vi "GetPositionDegreeInc.vi"(8 "error in (no error)":errorcluster, 10 "IncImpulsIn":dbl caption="Инкремент импульсов", 11 "StepMotor in":refnum<class "StepMotor.lvclass">) -> (0 "error out":errorcluster, 2 "IncImpulsOut":dbl caption="Инкремент импульсов", 3 "StepMotor out":refnum<class "StepMotor.lvclass">)   [LabVIEW 2010, in "StepMotor.lvclass"]
uses:
  StepMotor.lvclass
panel:
  out "RawValue":dbl
  out "Текущая позиция":dbl
  out "Предыдущая позиция":dbl
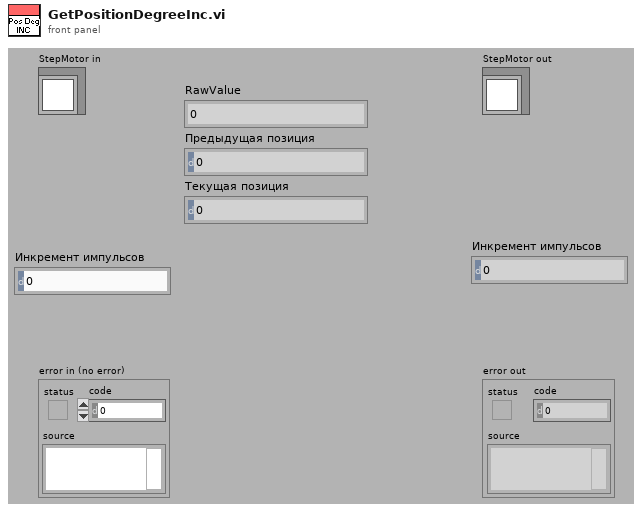
[diagram p1: front panel]
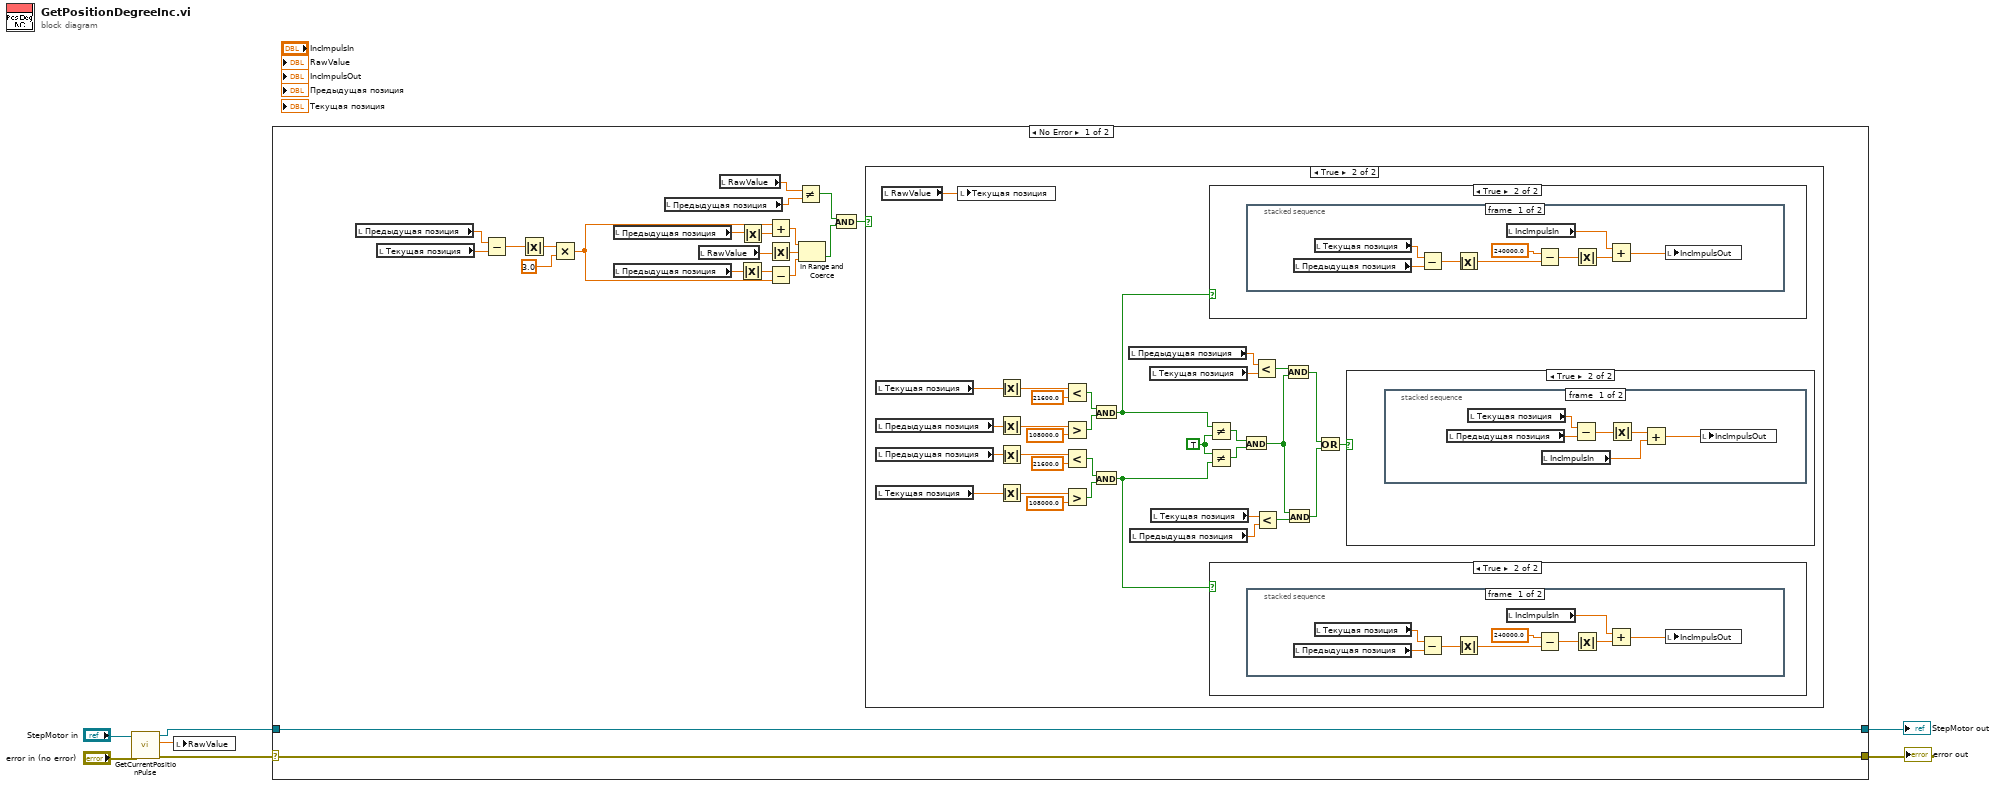
[diagram p0: block diagram]
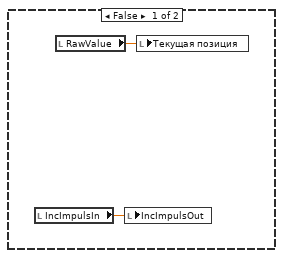
[diagram p2: hidden frame]
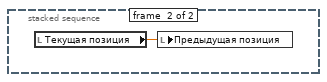
[diagram p4: hidden frame]
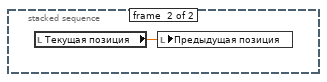
[diagram p6: hidden frame]
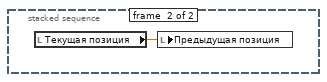
[diagram p8: hidden frame]
diagram:
  n1 = call-dynamic "GetCurrentPositionPulse.vi"("error in (no error)"="error in (no error)", "StepMotor in"="StepMotor in") -> ("error out"=w2:errorcluster, "Текущая позиция"=w5:dbl, "StepMotor out"=w1:refnum<class "StepMotor.lvclass">)  [unwired: 7 in]
  n2 = local write "RawValue"(w5) -> ()
  n3 = case shown="No Error" w2 {
    selector: w2 -> [w10 w91]
    tunnel: [w10 w91] -> w7
    tunnel: [w11 w90] -> w6
    tunnel: w1 -> [w11 w90]
    frame No Error {
      n4 = local read "Предыдущая позиция"() -> (w27:dbl)
      n5 = local read "Текущая позиция"() -> (w25:dbl)
      n6 = Subtract(x=w27, y=w25) -> (x-y=w24:dbl)
      n7 = Absolute Value(x=w24) -> (abs(x)=w22:dbl)
      n8 = Multiply(x=w22, y=3.0) -> (x*y=w28:dbl)
      n9 = local read "Предыдущая позиция"() -> (w18:dbl)
      n10 = local read "Предыдущая позиция"() -> (w17:dbl)
      n11 = local read "Предыдущая позиция"() -> (w26:dbl)
      n12 = local read "RawValue"() -> (w8:dbl)
      n13 = local read "RawValue"() -> (w9:dbl)
      n14 = Absolute Value(x=w17) -> (abs(x)=w16:dbl)
      n15 = Absolute Value(x=w18) -> (abs(x)=w19:dbl)
      n16 = Add(x=w28, y=w19) -> (x+y=w15:dbl)
      n17 = Absolute Value(x=w8) -> (abs(x)=w20:dbl)
      n18 = Subtract(x=w16, y=w28) -> (x-y=w14:dbl)
      n19 = Not Equal?(x=w9, y=w26) -> (x != y?=w13:bool)
      n20 = In Range and Coerce(upper limit=w15, x=w20, lower limit=w14) -> (In Range?=w12:bool)  [unwired: 1 out]
      n21 = Compound Arithmetic op=AND(w13, w12) -> (w23:bool)
      n22 = case shown="True" w23 {
        frame False {
          n23 = local read "IncImpulsIn"() -> (w29:dbl)
          n24 = local read "RawValue"() -> (w30:dbl)
          n25 = local write "IncImpulsOut"(w29) -> ()
          n26 = local write "Текущая позиция"(w30) -> ()
        }
        frame True {
          w54 = TRUE ("x")
          n27 = local read "Текущая позиция"() -> (w31:dbl)
          n28 = local read "Предыдущая позиция"() -> (w33:dbl)
          n29 = local read "Предыдущая позиция"() -> (w35:dbl)
          n30 = local read "Текущая позиция"() -> (w37:dbl)
          n31 = local read "RawValue"() -> (w39:dbl)
          n32 = local write "Текущая позиция"(w39) -> ()
          n33 = Absolute Value(x=w31) -> (abs(x)=w32:dbl)
          n34 = Absolute Value(x=w33) -> (abs(x)=w34:dbl)
          n35 = Absolute Value(x=w35) -> (abs(x)=w36:dbl)
          n36 = Absolute Value(x=w37) -> (abs(x)=w38:dbl)
          n37 = Less?(x=w32, y=21600.0) -> (x < y?=w57:bool)
          n38 = Greater?(x=w34, y=108000.0) -> (0:w58:bool)
          n39 = Less?(x=w36, y=21600.0) -> (x < y?=w56:bool)
          n40 = Greater?(x=w38, y=108000.0) -> (0:w55:bool)
          n41 = And(x=w57, y=w58) -> (x .and. y?=w43:bool)
          n42 = And(x=w56, y=w55) -> (x .and. y?=w42:bool)
          n43 = local read "Предыдущая позиция"() -> (w50:dbl)
          n44 = local read "Предыдущая позиция"() -> (w49:dbl)
          n45 = local read "Текущая позиция"() -> (w41:dbl)
          n46 = local read "Текущая позиция"() -> (w40:dbl)
          n47 = Not Equal?(x=w43, y=w54) -> (x != y?=w52:bool)
          n48 = Not Equal?(x=w54, y=w42) -> (x != y?=w53:bool)
          n49 = case shown="True" w43 {
            frame False {
            }
            frame True {
              n50 = stacked-sequence {
                frame #0 {
                  n51 = local read "Предыдущая позиция"() -> (w88:dbl)
                  n52 = local read "Текущая позиция"() -> (w80:dbl)
                  n53 = Subtract(x=w80, y=w88) -> (x-y=w87:dbl)
                  n54 = Absolute Value(x=w87) -> (abs(x)=w86:dbl)
                  n55 = local read "IncImpulsIn"() -> (w83:dbl)
                  n56 = Subtract(x=240000.0, y=w86) -> (x-y=w84:dbl)
                  n57 = Absolute Value(x=w84) -> (abs(x)=w81:dbl)
                  n58 = Add(x=w83, y=w81) -> (x+y=w82:dbl)
                  n59 = local write "IncImpulsOut"(w82) -> ()
                }
                frame #1 {
                  n60 = local read "Текущая позиция"() -> (w89:dbl)
                  n61 = local write "Предыдущая позиция"(w89) -> ()
                }
              }
            }
          }
          n62 = case shown="True" w42 {
            frame False {
            }
            frame True {
              n63 = stacked-sequence {
                frame #0 {
                  n64 = local read "Предыдущая позиция"() -> (w72:dbl)
                  n65 = local read "Текущая позиция"() -> (w70:dbl)
                  n66 = Subtract(x=w70, y=w72) -> (x-y=w73:dbl)
                  n67 = Absolute Value(x=w73) -> (abs(x)=w74:dbl)
                  n68 = local read "IncImpulsIn"() -> (w77:dbl)
                  n69 = Subtract(x=240000.0, y=w74) -> (x-y=w76:dbl)
                  n70 = Absolute Value(x=w76) -> (abs(x)=w78:dbl)
                  n71 = Add(x=w77, y=w78) -> (x+y=w71:dbl)
                  n72 = local write "IncImpulsOut"(w71) -> ()
                }
                frame #1 {
                  n73 = local read "Текущая позиция"() -> (w79:dbl)
                  n74 = local write "Предыдущая позиция"(w79) -> ()
                }
              }
            }
          }
          n75 = And(x=w52, y=w53) -> (x .and. y?=w51:bool)
          n76 = Less?(x=w50, y=w41) -> (x < y?=w47:bool)
          n77 = Less?(x=w40, y=w49) -> (x < y?=w48:bool)
          n78 = And(x=w47, y=w51) -> (x .and. y?=w46:bool)
          n79 = And(x=w51, y=w48) -> (x .and. y?=w45:bool)
          n80 = Or(x=w46, y=w45) -> (x .or. y?=w44:bool)
          n81 = case shown="True" w44 {
            frame False {
            }
            frame True {
              n82 = stacked-sequence {
                frame #0 {
                  n83 = local read "Предыдущая позиция"() -> (w68:dbl)
                  n84 = local read "Текущая позиция"() -> (w65:dbl)
                  n85 = local read "IncImpulsIn"() -> (w63:dbl)
                  n86 = Subtract(x=w65, y=w68) -> (x-y=w67:dbl)
                  n87 = Absolute Value(x=w67) -> (abs(x)=w66:dbl)
                  n88 = Add(x=w66, y=w63) -> (x+y=w64:dbl)
                  n89 = local write "IncImpulsOut"(w64) -> ()
                }
                frame #1 {
                  n90 = local read "Текущая позиция"() -> (w69:dbl)
                  n91 = local write "Предыдущая позиция"(w69) -> ()
                }
              }
            }
          }
        }
      }
    }
    frame Error {
    }
  }
  "error out" <- w7
  "StepMotor out" <- w6
